vi "Lex Symbolic Number.vi"(8 "error in (no error)":errorcluster, 11 "JSON Lexer in":refnum<class "JSON Lexer.lvclass">) -> (0 "error out":errorcluster, 1 "EOF":bool, 2 "Next State":T1=enum."Value", 3 "JSON Lexer out":refnum<class "JSON Lexer.lvclass">)   [LabVIEW 2013, in "JKI JSON Serialization.lvlib" / "JSON Lexer.lvclass"]
uses:
  JSON Lexer.lvclass
  JSON Lexer States.ctl
  JSON Token Type.ctl
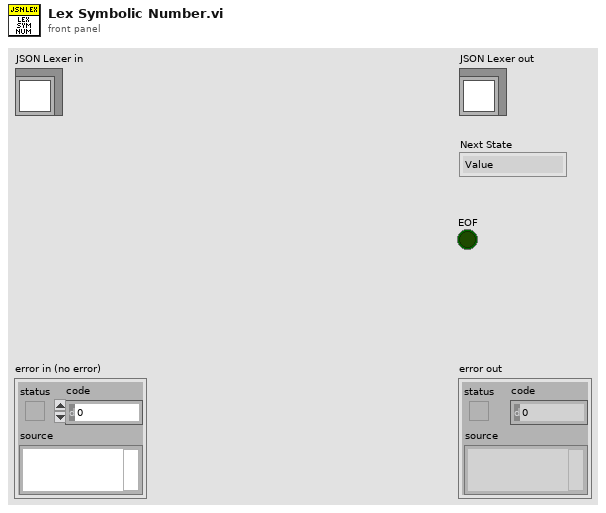
[diagram p1: front panel]
types:
  T1 = typedef "JKI JSON Serialization.lvlib/JSON Lexer.lvclass/JSON Lexer States.ctl" = enum16{"Undefined", "Value", "String", "Numeric", "Number", "Symbol", "Symbolic Number"}
  T2 = typedef "JKI JSON Serialization.lvlib/JSON Lexer.lvclass/JSON Token Type.ctl" = enum32{"unknown", "comma", "end-label", "begin-object", "end-object", "begin-array", "end-array", "quoted-string", "boolean", "exponential-number", "decimal-number", "integer-number", "special-number", "null", "symbol", "whitespace", "EOF"}
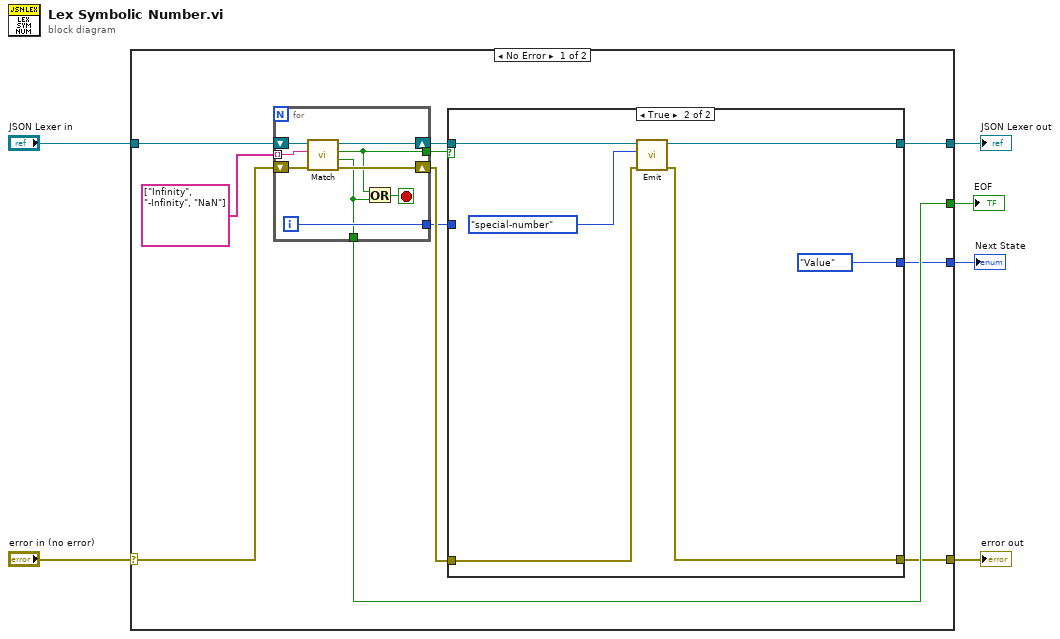
[diagram p0: block diagram]
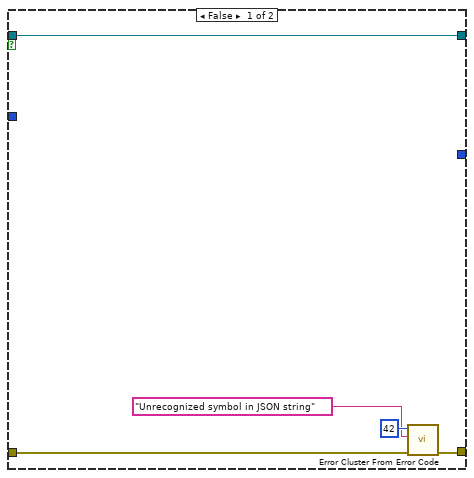
[diagram p2: hidden frame]
diagram:
  n1 = case shown="No Error" "error in (no error)" {
    selector: "error in (no error)" -> [w16 w39]
    tunnel: [w11 w39] -> w5
    tunnel: [w8 w38] -> w3
    tunnel: "JSON Lexer in" -> [w17 w38]
    tunnel: [w13 _] -> w2
    tunnel: [w7 _] -> w1
    frame No Error {
      n2 = for {
        shift-right: [w36] -> w10
        shift-left: w17 -> [w37]
        shift-right: [w33] -> w12
        shift-left: w16 -> [w34]
        tunnel: string[] ["Infinity", "-Infinity", "NaN"] -> [w32] mode=indexing
        tunnel: [w31] -> w9
        tunnel: [w30] -> w14
        tunnel: [w29] -> w13
        i -> [w31]
        stop <- w35 stop-if-true
        n3 = call "Match.vi"("error in (no error)"=w34, "Match String"=w32, "JSON Lexer in"=w37) -> ("error out"=w33:errorcluster, "EOF"=w29:bool, "Matched?"=w30:bool, "JSON Lexer out"=w36:refnum<class "JSON Lexer.lvclass">)  [unwired: 5 in]
        n4 = Or(x=w30, y=w29) -> (x .or. y?=w35:bool)
      }
      n5 = case shown="True" w14 {
        tunnel: w12 -> [w20 w26]
        tunnel: [w21 w25] -> w11
        tunnel: w10 -> [w22 w28]
        tunnel: w9 -> [_ _]
        tunnel: [w22 w27] -> w8
        tunnel: [_ JSON_Lexer_States."Value" ("JSON Lexer State")] -> w7
        frame False {
          n6 = call <vilib>:"Error Cluster From Error Code.vi"("error in (no error)"=w20, "error message (\"\")"="Unrecognized symbol in JSON string", "error code (0)"=42) -> ("error out"=w21:errorcluster)  [unwired: 6 in]
        }
        frame True {
          n7 = call "Emit.vi"("error in (no error)"=w26, "JSON Token Type"=JSON_Token_Type."special-number", "JSON Lexer in"=w28) -> ("error out"=w25:errorcluster, "JSON Lexer out"=w27:refnum<class "JSON Lexer.lvclass">)  [unwired: 7 in]
        }
      }
    }
    frame Error {
    }
  }
  "error out" <- w5
  "JSON Lexer out" <- w3
  "Next State" <- w1
  "EOF" <- w2
